vi "Configure Channel (Current).vi"(4 "Power Line Cycles (0)":i32, 5 "Voltage Limit (2.0 V)":dbl=2.0, 6 "Triggered Level (1.0 mA)":dbl=0.001, 7 "Current Range (0: 1 uA)":u16(ring) items=["1 uA", "10 uA", "100 uA", "1 mA", "10 mA", "120 mA"], 8 "error in (no error)":errorcluster, 9 "Output Level (1.0 mA)":dbl=0.001, 10 "Channel (1: Channel 1)":u16(ring)=1 items=["Channel 1"=1, "Channel 2"=2, "Channel 3"=3], 11 "VISA resource name":refnum<visa-resource-name>) -> (0 "error out":errorcluster, 3 "VISA resource name out":refnum<visa-resource-name>)   [LabVIEW 2018, in "Agilent U2722.lvlib"]
doc: "Configures the channel to output in source current mode."
uses:
  Agilent U2722.lvlib
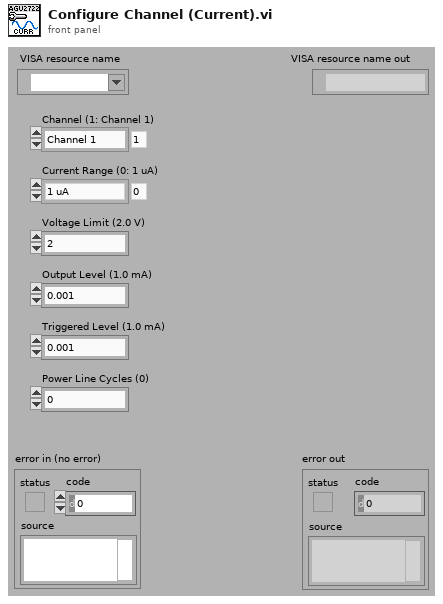
[diagram p1: front panel]
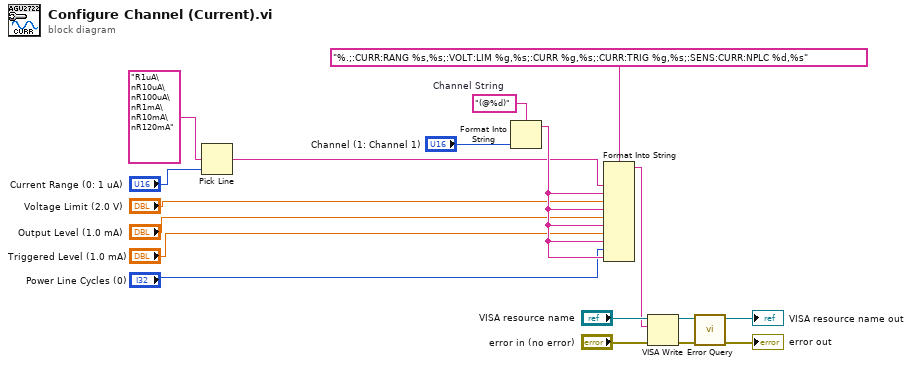
[diagram p0: block diagram]
diagram:
  w12 = "(@%d)"  # Channel String
  n1 = Pick Line(multi-line string="R1uA\nR10uA\nR100uA\nR1mA\nR10mA\nR120mA", line index="Current Range (0: 1 uA)") -> (output string=w1:string)  [unwired: 1 in]
  n2 = Format Into String(format string=w12, "Channel (1: Channel 1)") -> (resulting string=w10:string)  [unwired: 2 in, 1 out]
  n3 = Format Into String(format string="%.;:CURR:RANG %s,%s;:VOLT:LIM %g,%s;:CURR %g,%s;:CURR:TRIG %g,%s;:SENS:CURR:NPLC %d,%s", w1, w10, "Voltage Limit (2.0 V)", w10, "Output Level (1.0 mA)", w10, "Triggered Level (1.0 mA)", w10, "Power Line Cycles (0)", w10) -> (resulting string=w9:string)  [unwired: 2 in, 1 out]
  n4 = VISA Write(VISA resource name="VISA resource name", write buffer=w9, error in (no error)="error in (no error)") -> (VISA resource name out=w14:refnum<visa-resource-name>, error out=w13:errorcluster)  [unwired: 1 out]
  n5 = call "Error Query.vi"("error in (no error)"=w13, "VISA resource name"=w14) -> ("error out"=→"error out":errorcluster, "VISA resource name out"=→"VISA resource name out":refnum<visa-resource-name>)  [unwired: 6 in, 2 out]
